vi "Get PID.vi"(10 "Subsystem":string) -> (1 "PID Gains":T1, 3 "output range":cluster{"output high":dbl, "output low":dbl})   [LabVIEW 2015]
uses:
  <vilib>/Rock Robotics/Network Tables/NT Read Number.vi
panel:
  in  "output range":cluster{"output high":dbl, "output low":dbl}={"output high"=100.0, "output low"=-100.0} {"output low" format="%.2f"; "output high" format="%.2f"}
  in  "PID gains":T1={"proportional gain (Kc)"=1.0, "integral time (Ti, min)"=0.01, "derivative time (Td, min)"=0.0} {"derivative time (Td, min)" format="%.3f"; "integral time (Ti, min)" format="%.3f"; "proportional gain (Kc)" format="%.3f"}
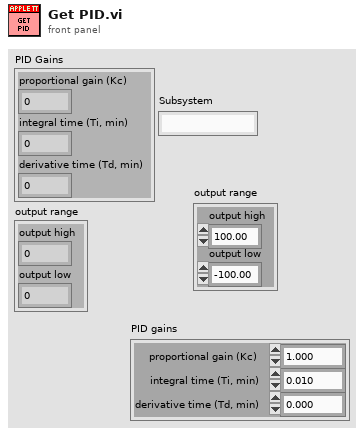
[diagram p1: front panel]
types:
  T1 = cluster{"proportional gain (Kc)":dbl, "integral time (Ti, min)":dbl, "derivative time (Td, min)":dbl}
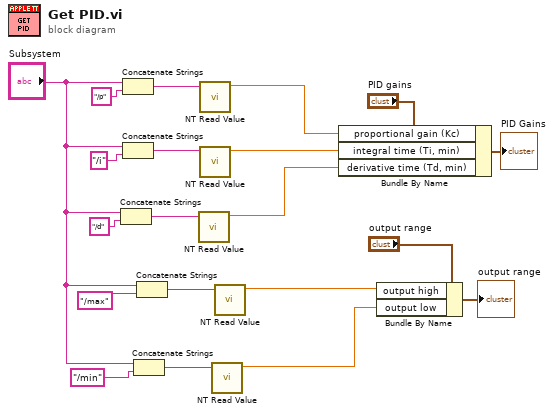
[diagram p0: block diagram]
diagram:
  n1 = Concatenate Strings("Subsystem", "/d") -> (w15:string)
  n2 = Concatenate Strings("Subsystem", "/p") -> (w19:string)
  n3 = Concatenate Strings("Subsystem", "/i") -> (w16:string)
  n4 = Concatenate Strings("Subsystem", "/min") -> (w12:string)
  n5 = Concatenate Strings("Subsystem", "/max") -> (w14:string)
  n6 = call-poly <vilib>:"NT Read Value.vi"("Name"=w15) -> ("Numeric"=w6:dbl)  [unwired: 9 in, 1 out]
  n7 = call-poly <vilib>:"NT Read Value.vi"("Name"=w19) -> ("Numeric"=w8:dbl)  [unwired: 9 in, 1 out]
  n8 = call-poly <vilib>:"NT Read Value.vi"("Name"=w16) -> ("Numeric"=w7:dbl)  [unwired: 9 in, 1 out]
  n9 = call-poly <vilib>:"NT Read Value.vi"("Name"=w12) -> ("Numeric"=w3:dbl)  [unwired: 9 in, 1 out]
  n10 = call-poly <vilib>:"NT Read Value.vi"("Name"=w14) -> ("Numeric"=w4:dbl)  [unwired: 9 in, 1 out]
  n11 = Bundle By Name(cluster="PID gains", "proportional gain (Kc)"=w8, "integral time (Ti, min)"=w7, "derivative time (Td, min)"=w6) -> (→"PID Gains":T1)
  n12 = Bundle By Name(cluster="output range", "output high"=w4, "output low"=w3) -> (→"output range":cluster{"output high":dbl, "output low":dbl})
